vi "TDS Base Initialize.vi"(8 "error in (no error)":errorcluster, 10 "InstSpecific":string, 11 "Address":string) -> (0 "error out":errorcluster)   [LabVIEW 2025, in "Interface Functions.lvlib"]
uses:
  Interface Functions.lvlib
panel:
  # "Base Initialize"
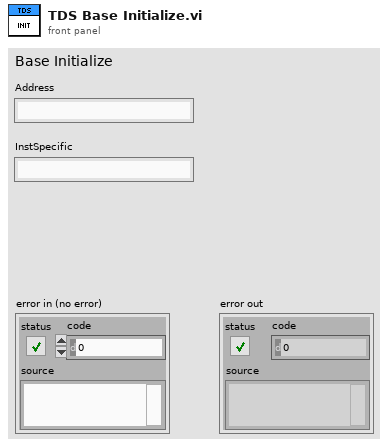
[diagram p1: front panel]
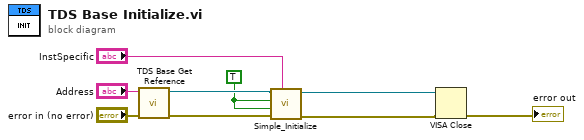
[diagram p0: block diagram]
diagram:
  w2 = TRUE ("ID Query (True)")
  n1 = call "TDS Base Get Reference.vi"("error in (no error)"="error in (no error)", "Address"="Address") -> ("error out"=w6:errorcluster, "Reference"=w7:refnum<visa-resource-name>)  [unwired: 8 in]
  n2 = call "Simple_Initialize.vi"("PwrSns Model RegEx"="InstSpecific", "error in (no error)"=w6, "Reset (True)"=w2, "ID Query (True)"=w2, "VISA resource name"=w7) -> ("error out"=w5:errorcluster, "VISA resource name out"=w3:refnum<visa-resource-name>)  [unwired: 5 in]
  n3 = VISA Close(VISA resource name=w3, error in (no error)=w5) -> (error out=→"error out":errorcluster)
